vi "Load Icon.vi"(8 "error in (no error)":errorcluster, 9 "Icon path True":path, 10 "Icon path False":path, 11 "Control in":refnum<class "Control.lvclass">) -> (0 "error out":errorcluster, 3 "Control out":refnum<class "Control.lvclass">)   [LabVIEW 2013, in "Control.lvclass"]
doc: "Load an icon for the control object."
uses:
  Control.lvclass
  Control.lvclass/Control.ctl
  <userlib>/_OpenG.lib/file/file.llb/Strip Path - Traditional__ogtk.vi
  <userlib>/_OpenG.lib/file/file.llb/Strip Path Extension - String__ogtk.vi
  <userlib>/BitMan/BitMap class/BitMap.lvclass
  <userlib>/BitMan/Built-in Filters class/Built-in Filters.lvclass
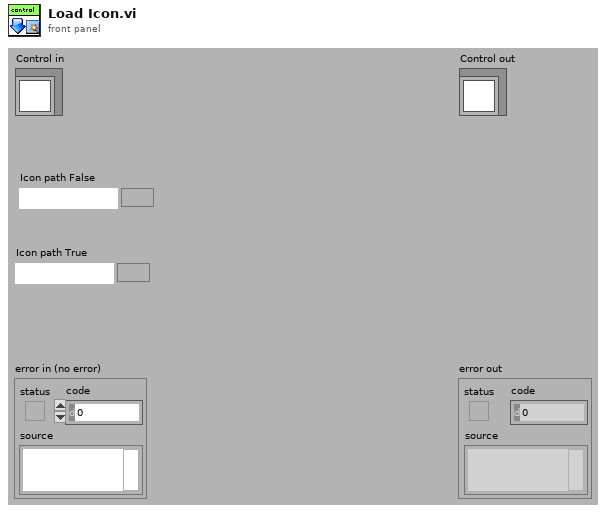
[diagram p1: front panel]
types:
  T1 = typedef "imagedata.ctl" = cluster{"image type":i32, "image depth":i32, "image":u8[], "mask":u8[], "colors":u32[], "Rectangle":cluster{"left":i16, "top":i16, "right":i16, "bottom":i16}}
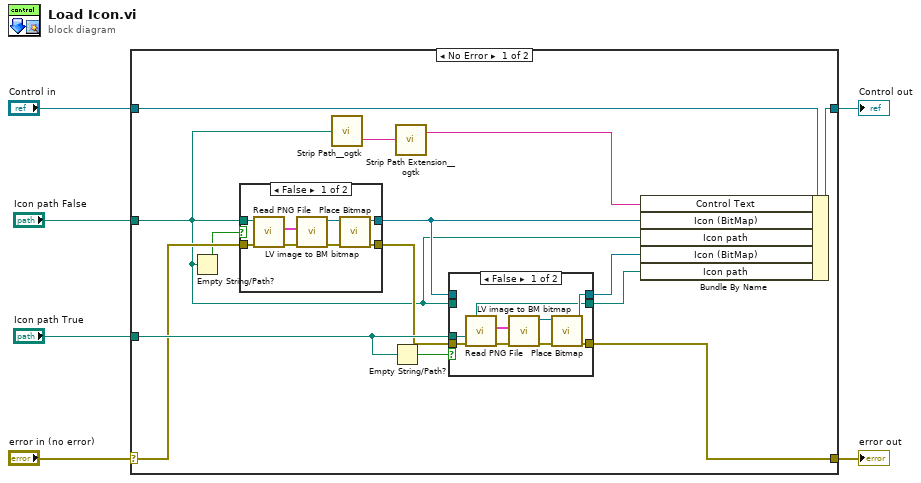
[diagram p0: block diagram]
diagram:
  n1 = case shown="No Error" "error in (no error)" {
    selector: "error in (no error)" -> [w10 w42]
    tunnel: [w9 w42] -> w5
    tunnel: [w20 w41] -> w4
    tunnel: "Control in" -> [w17 w41]
    tunnel: "Icon path False" -> [w8 _]
    tunnel: "Icon path True" -> [w15 _]
    frame No Error {
      n2 = Empty String/Path?(string/path=w8) -> (empty?=w7:bool)
      n3 = case shown="False" w7 {
        tunnel: [w24 _] -> w14
        tunnel: [w23 w29] -> w11
        tunnel: w10 -> [w22 w29]
        tunnel: w8 -> [w21 _]
        frame False {
          n4 = call <vilib>:"Read PNG File.vi"("error in (no error)"=w22, "path to PNG file"=w21) -> ("error out"=w26:errorcluster, "image data"=w25:T1)  [unwired: 8 out]
          n5 = call <userlib>:"LV image to BM bitmap.vi"("error in (no error)"=w26, "LV image data"=w25) -> ("error out"=w27:errorcluster, "BitMap out"=w28:refnum<class "BitMap.lvclass">)  [unwired: 2 in, 6 out]
          n6 = call <userlib>:"Place Bitmap.vi"("error in (no error)"=w27, "Bitmap in (optional)"=w28) -> ("error out"=w23:errorcluster, "Bitmap out"=w24:refnum<class "BitMap.lvclass">)  [unwired: 4 in, 4 out]
        }
        frame True {
        }
      }
      n7 = call-poly <userlib>:"Strip Path__ogtk.vi"("path"=w8) -> ("name"=w19:string)  [unwired: 1 out]
      n8 = Empty String/Path?(string/path=w15) -> (empty?=w16:bool)
      n9 = call-poly <userlib>:"Strip Path Extension__ogtk.vi"("path"=w19) -> ("root"=w18:string)  [unwired: 1 out]
      n10 = case shown="False" w16 {
        tunnel: w15 -> [w32 _]
        tunnel: w14 -> [_ w40]
        tunnel: [w33 w40] -> w13
        tunnel: w8 -> [_ w39]
        tunnel: [w32 w39] -> w12
        tunnel: w11 -> [w31 w38]
        tunnel: [w30 w38] -> w9
        frame False {
          n11 = call <vilib>:"Read PNG File.vi"("error in (no error)"=w31, "path to PNG file"=w32) -> ("error out"=w36:errorcluster, "image data"=w37:T1)  [unwired: 8 out]
          n12 = call <userlib>:"LV image to BM bitmap.vi"("error in (no error)"=w36, "LV image data"=w37) -> ("error out"=w35:errorcluster, "BitMap out"=w34:refnum<class "BitMap.lvclass">)  [unwired: 2 in, 6 out]
          n13 = call <userlib>:"Place Bitmap.vi"("error in (no error)"=w35, "Bitmap in (optional)"=w34) -> ("error out"=w30:errorcluster, "Bitmap out"=w33:refnum<class "BitMap.lvclass">)  [unwired: 4 in, 4 out]
        }
        frame True {
        }
      }
      n14 = Bundle By Name(cluster=w17, "Control Text"=w18, "Icon (BitMap)"=w14, "Icon path"=w8, "Icon (BitMap)"=w13, "Icon path"=w12) -> (w20:refnum<class "Control.lvclass">)
    }
    frame Error {
    }
  }
  "error out" <- w5
  "Control out" <- w4
